vi "Bass Only Live.vi"() -> ()   [LabVIEW 2009]
uses:
  <vilib>/vision/Image Controls.llb/IMAQ Image.ctl
  <vilib>/Instr/_visa.llb/VISA Configure Serial Port (Instr).vi
  <vilib>/userDefined/High Color/IMAQdx.ctl
  <vilib>/Analysis/3filter.llb/Filter Passband Type.ctl
  <vilib>/Analysis/3filter.llb/Butterworth Filter (DBL).vi
  <vilib>/vision/NI_Vision_Development_Module.lvlib
  <vilib>/Analysis/NI_AALBase.lvlib
  <vilib>/vision/driver/NI_Vision_Acquisition_Software.lvlib
panel:
  in  "Orange Guitar":T1={"Global Rectangle"=[220, 302, 227, 392], "Contours"=[{"ID"=enum."External", "Type"=2, "Coordinates"=[226, 391, 220, 302]}]} {"Contours"."Type" items=["No Selection", "Point", "Line", "Rectangle", "Oval", "Polygon", "Freehand Region", "Annulus", "Unused2", "Unused3", "Broken Line", "Freehand Line", "Rotated Rectangle"]}
  in  "Blue Guitar":T1={"Global Rectangle"=[192, 292, 199, 386], "Contours"=[{"ID"=enum."External", "Type"=2, "Coordinates"=[192, 385, 198, 292]}]} {"Contours"."Type" items=["No Selection", "Point", "Line", "Rectangle", "Oval", "Polygon", "Freehand Region", "Annulus", "Unused2", "Unused3", "Broken Line", "Freehand Line", "Rotated Rectangle"]}
  out "Orange Guitar":dbl[](graph)
  out "Orange Guitar LED":bool
  in  "sampling 8":dbl=1.0 format="%0.2f"
  in  "high 9":dbl=60.0 format="%0.2f"
  in  "low  8":dbl=0.12500000000000006 format="%0.4f"
  out "Orange Guitar":T1={"Global Rectangle"=[300, 297, 320, 380], "Contours"=[{"ID"=enum."External", "Type"=2, "Coordinates"=[300, 379, 319, 297]}]} {"Contours"."Type" items=["No Selection", "Point", "Line", "Rectangle", "Oval", "Polygon", "Freehand Region", "Annulus", "Unused2", "Unused3", "Broken Line", "Freehand Line", "Rotated Rectangle"]}
  in  "Green Guitar":T1={"Global Rectangle"=[100, 292, 131, 371], "Contours"=[{"ID"=enum."External", "Type"=2, "Coordinates"=[100, 370, 130, 292]}]} {"Contours"."Type" items=["No Selection", "Point", "Line", "Rectangle", "Oval", "Polygon", "Freehand Region", "Annulus", "Unused2", "Unused3", "Broken Line", "Freehand Line", "Rotated Rectangle"]}
  in  "Red Guitar":T1={"Global Rectangle"=[129, 294, 154, 376], "Contours"=[{"ID"=enum."External", "Type"=2, "Coordinates"=[129, 375, 153, 294]}]} {"Contours"."Type" items=["No Selection", "Point", "Line", "Rectangle", "Oval", "Polygon", "Freehand Region", "Annulus", "Unused2", "Unused3", "Broken Line", "Freehand Line", "Rotated Rectangle"]}
  in  "Yellow Guitar":T1={"Global Rectangle"=[160, 295, 175, 378], "Contours"=[{"ID"=enum."External", "Type"=2, "Coordinates"=[160, 377, 174, 295]}]} {"Contours"."Type" items=["No Selection", "Point", "Line", "Rectangle", "Oval", "Polygon", "Freehand Region", "Annulus", "Unused2", "Unused3", "Broken Line", "Freehand Line", "Rotated Rectangle"]}
  in  "sampling  8":dbl=1.0 format="%0.2f"
  in  "high 8":dbl=60.0 format="%0.2f"
  out "Blue Guitar":dbl[](graph)
  in  "low 2":dbl=0.12500000000000006 format="%0.4f"
  out "Yellow Guitar":dbl[](graph)
  out "Yellow Guitar LED":bool
  in  "sampling 7":dbl=1.0 format="%0.2f"
  in  "high 7":dbl=60.0 format="%0.2f"
  in  "low  7":dbl=0.12500000000000006 format="%0.4f"
  out "Yellow Guitar":T1={"Global Rectangle"=[243, 262, 261, 384], "Contours"=[{"ID"=enum."External", "Type"=2, "Coordinates"=[260, 383, 243, 262]}]} {"Contours"."Type" items=["No Selection", "Point", "Line", "Rectangle", "Oval", "Polygon", "Freehand Region", "Annulus", "Unused2", "Unused3", "Broken Line", "Freehand Line", "Rotated Rectangle"]}
  out "Blue Guitar":T1={"Global Rectangle"=[168, 264, 180, 378], "Contours"=[{"ID"=enum."External", "Type"=2, "Coordinates"=[168, 377, 179, 264]}]} {"Contours"."Type" items=["No Selection", "Point", "Line", "Rectangle", "Oval", "Polygon", "Freehand Region", "Annulus", "Unused2", "Unused3", "Broken Line", "Freehand Line", "Rotated Rectangle"]}
  out "Green Guitar":dbl[](graph)
  out "Green Guitar LED":bool
  in  "sampling 6":dbl=1.0 format="%0.2f"
  in  "high 6":dbl=60.0 format="%0.2f"
  in  "low  6":dbl=0.12500000000000006 format="%0.4f"
  out "Green Guitar":T1={"Global Rectangle"=[406, 309, 423, 383], "Contours"=[{"ID"=enum."External", "Type"=2, "Coordinates"=[422, 382, 406, 309]}]} {"Contours"."Type" items=["No Selection", "Point", "Line", "Rectangle", "Oval", "Polygon", "Freehand Region", "Annulus", "Unused2", "Unused3", "Broken Line", "Freehand Line", "Rotated Rectangle"]}
  out "Red Guitar":dbl[](graph)
  out "Red Guitar LED":bool
  in  "sampling 5":dbl=1.0 format="%0.2f"
  in  "high 5":dbl=60.0 format="%0.2f"
  in  "low  5":dbl=0.12500000000000006 format="%0.4f"
  out "Red Guitar":T1={"Global Rectangle"=[300, 297, 320, 380], "Contours"=[{"ID"=enum."External", "Type"=2, "Coordinates"=[300, 379, 319, 297]}]} {"Contours"."Type" items=["No Selection", "Point", "Line", "Rectangle", "Oval", "Polygon", "Freehand Region", "Annulus", "Unused2", "Unused3", "Broken Line", "Freehand Line", "Rotated Rectangle"]}
  out "Blue Guitar LED":bool
  in  "Mask":T1 {"Contours"."Type" items=["No Selection", "Point", "Line", "Rectangle", "Oval", "Polygon", "Freehand Region", "Annulus", "Unused2", "Unused3", "Broken Line", "Freehand Line", "Rotated Rectangle"]}
  out "Image 2":T2(plugin-control)
  out "Red Line":T1={"Global Rectangle"=[300, 297, 320, 380], "Contours"=[{"ID"=enum."External", "Type"=2, "Coordinates"=[300, 379, 319, 297]}]} {"Contours"."Type" items=["No Selection", "Point", "Line", "Rectangle", "Oval", "Polygon", "Freehand Region", "Annulus", "Unused2", "Unused3", "Broken Line", "Freehand Line", "Rotated Rectangle"]}
  in  "Red Line":T1={"Global Rectangle"=[300, 297, 320, 380], "Contours"=[{"ID"=enum."External", "Type"=2, "Coordinates"=[300, 379, 319, 297]}]} {"Contours"."Type" items=["No Selection", "Point", "Line", "Rectangle", "Oval", "Polygon", "Freehand Region", "Annulus", "Unused2", "Unused3", "Broken Line", "Freehand Line", "Rotated Rectangle"]}
  out "Waveform Red":dbl[](graph)
  out "LED Red":bool
  in  "sampling 4":dbl=1.0 format="%0.2f"
  in  "high 4":dbl=60.0 format="%0.2f"
  in  "low  4":dbl=0.12500000000000006 format="%0.4f"
  out "Green Line":T1={"Global Rectangle"=[406, 309, 423, 383], "Contours"=[{"ID"=enum."External", "Type"=2, "Coordinates"=[422, 382, 406, 309]}]} {"Contours"."Type" items=["No Selection", "Point", "Line", "Rectangle", "Oval", "Polygon", "Freehand Region", "Annulus", "Unused2", "Unused3", "Broken Line", "Freehand Line", "Rotated Rectangle"]}
  in  "Blue Line":T1={"Global Rectangle"=[374, 278, 383, 377], "Contours"=[{"ID"=enum."External", "Type"=2, "Coordinates"=[382, 376, 374, 278]}]} {"Contours"."Type" items=["No Selection", "Point", "Line", "Rectangle", "Oval", "Polygon", "Freehand Region", "Annulus", "Unused2", "Unused3", "Broken Line", "Freehand Line", "Rotated Rectangle"]}
  in  "Green Line":T1={"Global Rectangle"=[406, 309, 423, 383], "Contours"=[{"ID"=enum."External", "Type"=2, "Coordinates"=[422, 382, 406, 309]}]} {"Contours"."Type" items=["No Selection", "Point", "Line", "Rectangle", "Oval", "Polygon", "Freehand Region", "Annulus", "Unused2", "Unused3", "Broken Line", "Freehand Line", "Rotated Rectangle"]}
  in  "low  3":dbl=0.12500000000000006 format="%0.4f"
  out "Waveform Green":dbl[](graph)
  out "LED Green":bool
  in  "sampling 3":dbl=1.0 format="%0.2f"
  in  "high 3":dbl=60.0 format="%0.2f"
  in  "Yellow Line":T1={"Global Rectangle"=[342, 292, 349, 377], "Contours"=[{"ID"=enum."External", "Type"=2, "Coordinates"=[342, 376, 348, 292]}]} {"Contours"."Type" items=["No Selection", "Point", "Line", "Rectangle", "Oval", "Polygon", "Freehand Region", "Annulus", "Unused2", "Unused3", "Broken Line", "Freehand Line", "Rotated Rectangle"]}
  out "Blue Line":T1={"Global Rectangle"=[168, 264, 180, 378], "Contours"=[{"ID"=enum."External", "Type"=2, "Coordinates"=[168, 377, 179, 264]}]} {"Contours"."Type" items=["No Selection", "Point", "Line", "Rectangle", "Oval", "Polygon", "Freehand Region", "Annulus", "Unused2", "Unused3", "Broken Line", "Freehand Line", "Rotated Rectangle"]}
  out "cluster":T3
  in  "baud rate (9600)":u32=9600
  in  "VISA resource name":refnum<visa-resource-name>
  out "number":u8
  out "decimal integer string":string
  out "Image Dst Out":T2
  out "Yellow Line":T1={"Global Rectangle"=[243, 262, 261, 384], "Contours"=[{"ID"=enum."External", "Type"=2, "Coordinates"=[260, 383, 243, 262]}]} {"Contours"."Type" items=["No Selection", "Point", "Line", "Rectangle", "Oval", "Polygon", "Freehand Region", "Annulus", "Unused2", "Unused3", "Broken Line", "Freehand Line", "Rotated Rectangle"]}
  in  "low  2":dbl=0.12500000000000006 format="%0.4f"
  in  "high 2":dbl=60.0 format="%0.2f"
  in  "sampling 2":dbl=1.0 format="%0.2f"
  out "LED Yellow":bool
  out "Waveform Yellow":dbl[](graph)
  in  "playtime":dbl=30.0
  out "Frame Number":i32
  in  "Frame Start":i32=2400
  out "Blue Drum":bool
  in  "low":dbl=0.12500000000000006 format="%0.4f"
  out "Blue Drum":dbl[](graph)
  in  "high":dbl=60.0 format="%0.2f"
  in  "sampling":dbl=1.0 format="%0.2f"
  in  "stop":bool
  # "BLUE"
  # "YELLOW"
  # "GREEN"
  # "RED"
  # "Drums"
  # "Guitar"
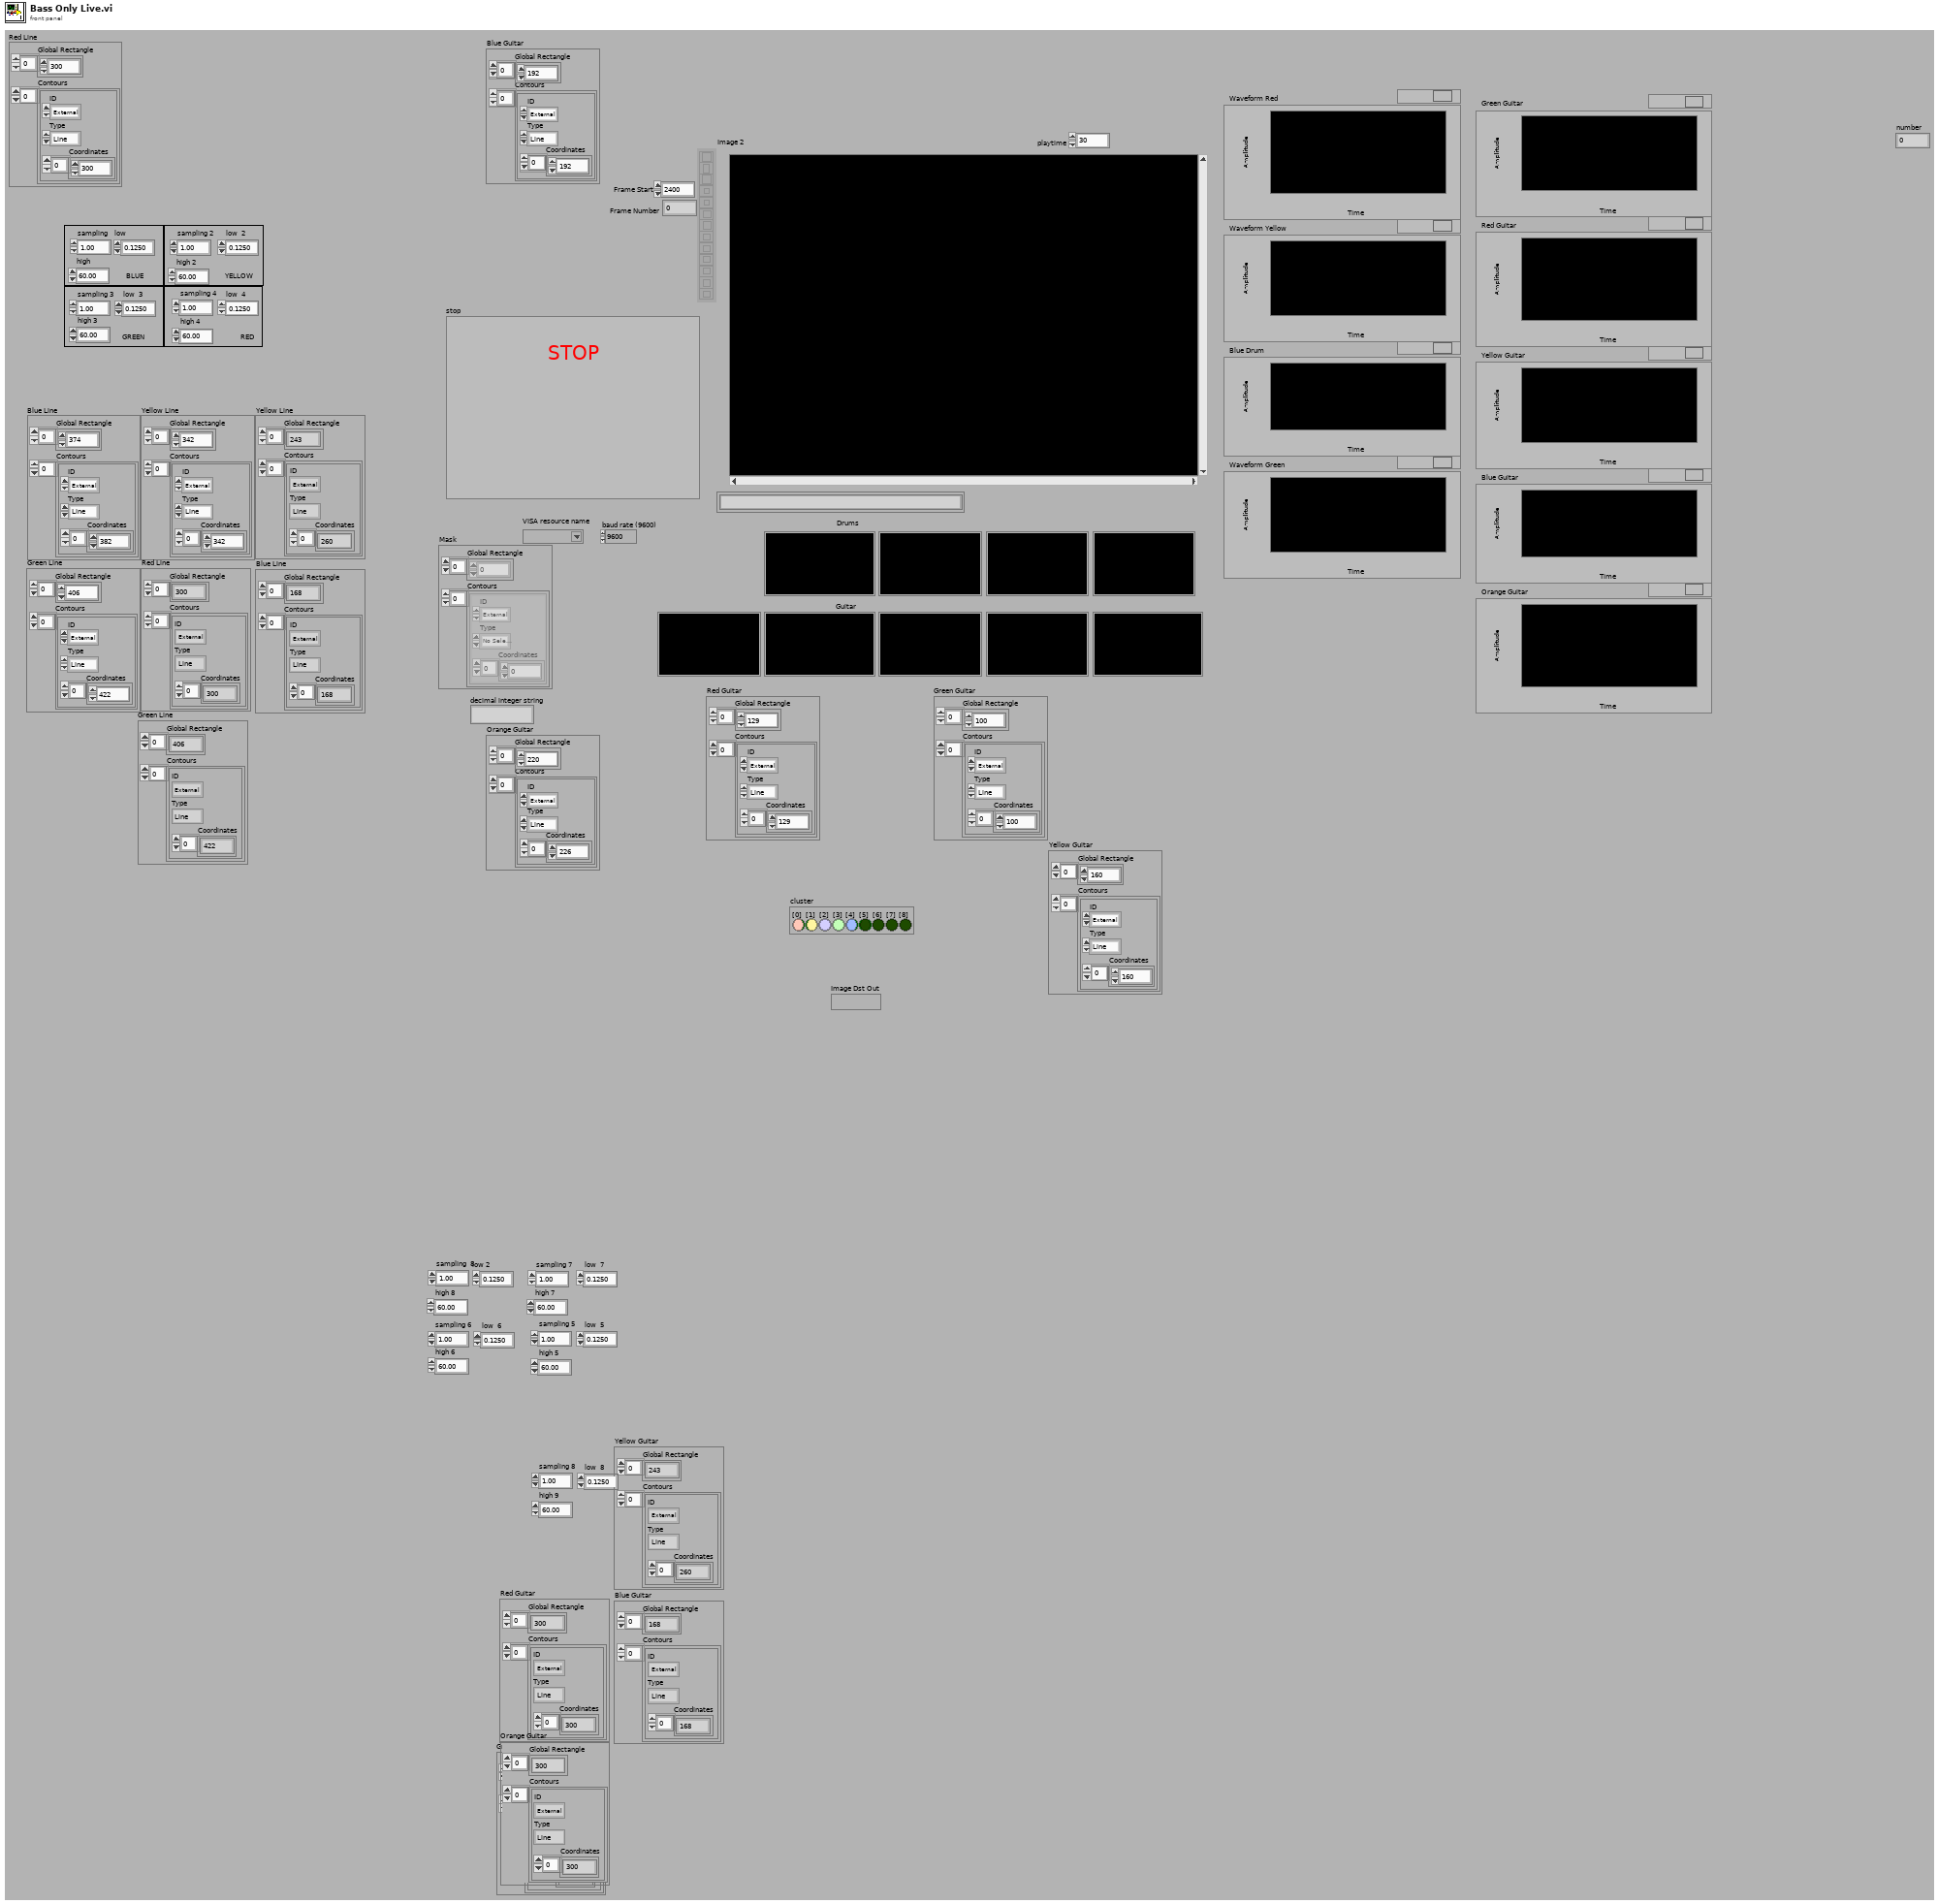
[diagram p1: front panel]
types:
  T1 = cluster{"Global Rectangle":i32[], "Contours":cluster{"ID":enum32{"External", "Internal"}, "Type":u32, "Coordinates":i32[]}[]}
  T2 = typedef "IMAQ Image.ctl" = refnum<image>
  T3 = cluster{"[0]":bool, "[1]":bool, "[2]":bool, "[3]":bool, "[4]":bool, "[5]":bool, "[6]":bool, "[7]":bool, "[8]":bool}
  T4 = typedef "IMAQdx.ctl" = refnum<k21>
  T5 = typedef "NI_AALBase.lvlib/Filter Passband Type.ctl" = enum32{"Lowpass", "Highpass", "Bandpass", "Bandstop"}
  T6 = cluster{"Left":i32, "Top":i32, "Right":i32, "Bottom":i32}
  T7 = typedef "Image Type" = u32
  T8 = cluster{"ID":enum32{"External", "Internal"}, "Type":u32, "Coordinates":i32[]}[]
  T9 = cluster{"ID":enum32{"External", "Internal"}, "Type":u32, "Coordinates":i32[]}
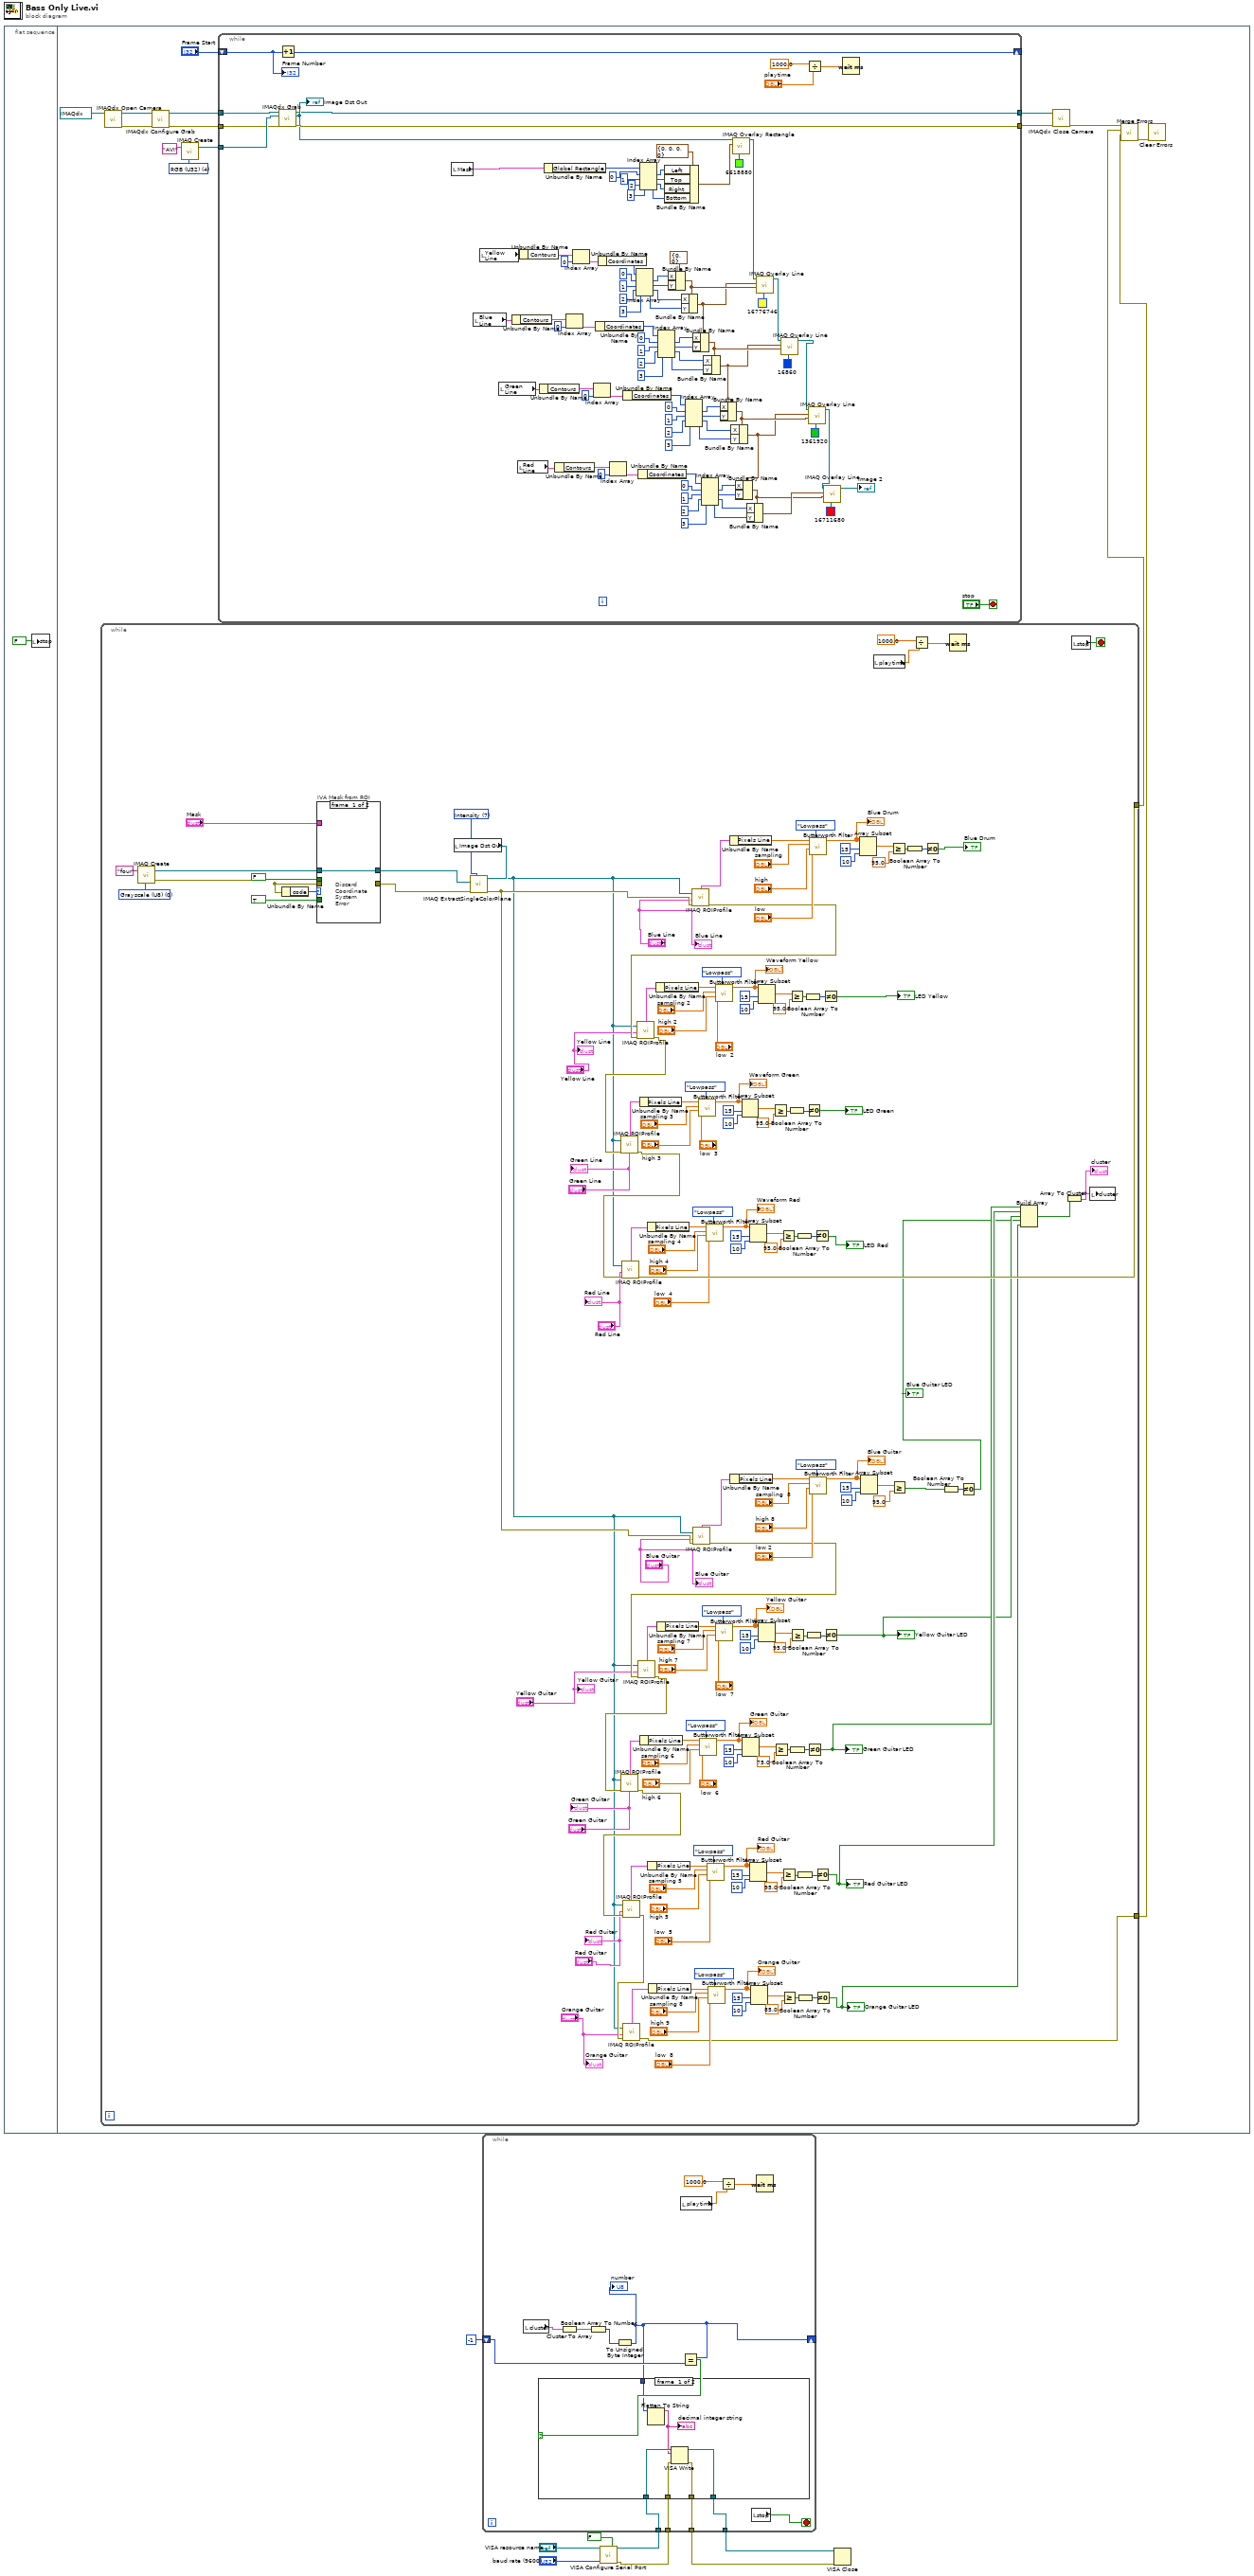
[diagram p0: block diagram]
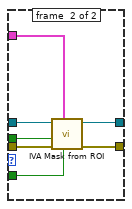
[diagram p3: hidden frame]
diagram:
  n1 = flat-sequence {
    frame #0 {
      n2 = local write "stop"(FALSE ("stop")) -> ()
    }
    frame #1 {
      w22 = T7 4 items=["Grayscale (U8)", "Grayscale (I16)", "Grayscale (SGL)", "Complex (CSG)", "RGB (U32)", "HSL (U32)", "RGB (U64)", "Grayscale (U16)"] ("Image Type")
      n3 = while {
        tunnel: [w172] -> w19
        tunnel: [w39] -> w18
        stop <- w187 stop-if-true
        w182 = T7 0 items=["Grayscale (U8)", "Grayscale (I16)", "Grayscale (SGL)", "Complex (CSG)", "RGB (U32)", "HSL (U32)", "RGB (U64)", "Grayscale (U16)"] ("Image Type")
        w188 = 7 items=["Red", "Green", "Blue", "Hue", "Saturation", "Luminance", "Value", "Intensity"] ("Color Plane")
        n4 = call "IMAQ Create"("Image Name"="four", "Image Type"=w182) -> ("New Image"=w175:T2, "error out"=w176:errorcluster)  [unwired: 3 in]
        n5 = Unbundle By Name(w176) -> ("code"=w180:i32)
        n6 = case "IVA Mask from ROI" shown="Default" w180 {
          tunnel: "Mask" -> [_ w196]
          tunnel: TRUE ("Shrink") -> [_ w195]
          tunnel: w175 -> [w189 w194]
          tunnel: w176 -> [_ w193]
          tunnel: [_ w192] -> w177
          tunnel: [w189 w191] -> w173
          tunnel: FALSE ("Out / In") -> [_ w190]
          frame #0 {
            # "Discard\nCoordinate\nSystem\nError"
          }
          frame #1 {
            n7 = call <vilib>:"IVA Mask from ROI.vi"("Shrink"=w195, "ROI Descriptor"=w196, "error in (no error)"=w193, "Out / In"=w190, "Image Src"=w194) -> ("error out"=w192:errorcluster, "Image Out"=w191:T2)  [unwired: 5 out]
          }
        }
        n8 = local read "Image Dst Out"() -> (w183:T2)
        n9 = call "IMAQ ExtractSingleColorPlane"("Color Plane"=w188, "error in (no error)"=w177, "Image Dst"=w173, "Image Src"=w183) -> ("error out"=w171:errorcluster, "Image Dst Out"=w38:T2)  [unwired: 6 out]
        n10 = call "IMAQ ROIProfile"("error in (no error)"=w171, "ROI Descriptor"="Blue Line", "Image"=w38) -> ("error out"=w146:errorcluster, "ROI Graph"=w145:cluster{"x0":sgl, "dx":sgl, "Pixels Line":sgl[]})  [unwired: 4 out]
        n11 = call "IMAQ ROIProfile"("error in (no error)"=w146, "ROI Descriptor"="Yellow Line", "Image"=w38) -> ("error out"=w113:errorcluster, "ROI Graph"=w149:cluster{"x0":sgl, "dx":sgl, "Pixels Line":sgl[]})  [unwired: 4 out]
        n12 = call "IMAQ ROIProfile"("error in (no error)"=w113, "ROI Descriptor"="Green Line", "Image"=w38) -> ("error out"=w116:errorcluster, "ROI Graph"=w143:cluster{"x0":sgl, "dx":sgl, "Pixels Line":sgl[]})  [unwired: 4 out]
        n13 = call "IMAQ ROIProfile"("error in (no error)"=w116, "ROI Descriptor"="Red Line", "Image"=w38) -> ("error out"=w172:errorcluster, "ROI Graph"=w118:cluster{"x0":sgl, "dx":sgl, "Pixels Line":sgl[]})  [unwired: 4 out]
        n14 = Unbundle By Name(w143) -> ("Pixels Line"=w140:sgl[])
        n15 = Unbundle By Name(w118) -> ("Pixels Line"=w121:sgl[])
        n16 = Unbundle By Name(w149) -> ("Pixels Line"=w152:sgl[])
        n17 = call "IMAQ ROIProfile"("error in (no error)"=w171, "ROI Descriptor"="Blue Guitar", "Image"=w38) -> ("error out"=w87:errorcluster, "ROI Graph"=w86:cluster{"x0":sgl, "dx":sgl, "Pixels Line":sgl[]})  [unwired: 4 out]
        n18 = call "IMAQ ROIProfile"("error in (no error)"=w87, "ROI Descriptor"="Yellow Guitar", "Image"=w38) -> ("error out"=w57:errorcluster, "ROI Graph"=w90:cluster{"x0":sgl, "dx":sgl, "Pixels Line":sgl[]})  [unwired: 4 out]
        n19 = call "IMAQ ROIProfile"("error in (no error)"=w57, "ROI Descriptor"="Green Guitar", "Image"=w38) -> ("error out"=w58:errorcluster, "ROI Graph"=w84:cluster{"x0":sgl, "dx":sgl, "Pixels Line":sgl[]})  [unwired: 4 out]
        n20 = call "IMAQ ROIProfile"("error in (no error)"=w58, "ROI Descriptor"="Red Guitar", "Image"=w38) -> ("error out"=w40:errorcluster, "ROI Graph"=w60:cluster{"x0":sgl, "dx":sgl, "Pixels Line":sgl[]})  [unwired: 4 out]
        n21 = call "IMAQ ROIProfile"("error in (no error)"=w40, "ROI Descriptor"="Orange Guitar", "Image"=w38) -> ("error out"=w39:errorcluster, "ROI Graph"=w52:cluster{"x0":sgl, "dx":sgl, "Pixels Line":sgl[]})  [unwired: 4 out]
        n22 = Unbundle By Name(w84) -> ("Pixels Line"=w81:sgl[])
        n23 = Unbundle By Name(w60) -> ("Pixels Line"=w63:sgl[])
        n24 = Unbundle By Name(w52) -> ("Pixels Line"=w49:sgl[])
        n25 = Unbundle By Name(w90) -> ("Pixels Line"=w93:sgl[])
        n26 = call-poly <vilib>:"Butterworth Filter.vi"("filter type"=Filter_Passband_Type."Lowpass", "low cutoff freq: fl"="low  3", "high cutoff freq: fh"="high 3", "sampling freq: fs"="sampling 3", "X"=w140) -> ("Filtered X"=w144:dbl[])  [unwired: 3 in, 1 out]
        "Waveform Green" <- w144
        n27 = call-poly <vilib>:"Butterworth Filter.vi"("filter type"=Filter_Passband_Type."Lowpass", "low cutoff freq: fl"="low  6", "high cutoff freq: fh"="high 6", "sampling freq: fs"="sampling 6", "X"=w81) -> ("Filtered X"=w85:dbl[])  [unwired: 3 in, 1 out]
        "Green Guitar" <- w85
        n28 = call-poly <vilib>:"Butterworth Filter.vi"("filter type"=Filter_Passband_Type."Lowpass", "low cutoff freq: fl"="low  4", "high cutoff freq: fh"="high 4", "sampling freq: fs"="sampling 4", "X"=w121) -> ("Filtered X"=w117:dbl[])  [unwired: 3 in, 1 out]
        "Waveform Red" <- w117
        n29 = call-poly <vilib>:"Butterworth Filter.vi"("filter type"=Filter_Passband_Type."Lowpass", "low cutoff freq: fl"="low  5", "high cutoff freq: fh"="high 5", "sampling freq: fs"="sampling 5", "X"=w63) -> ("Filtered X"=w59:dbl[])  [unwired: 3 in, 1 out]
        "Red Guitar" <- w59
        n30 = call-poly <vilib>:"Butterworth Filter.vi"("filter type"=Filter_Passband_Type."Lowpass", "low cutoff freq: fl"="low  8", "high cutoff freq: fh"="high 9", "sampling freq: fs"="sampling 8", "X"=w49) -> ("Filtered X"=w53:dbl[])  [unwired: 3 in, 1 out]
        "Orange Guitar" <- w53
        n31 = call-poly <vilib>:"Butterworth Filter.vi"("filter type"=Filter_Passband_Type."Lowpass", "low cutoff freq: fl"="low  2", "high cutoff freq: fh"="high 2", "sampling freq: fs"="sampling 2", "X"=w152) -> ("Filtered X"=w148:dbl[])  [unwired: 3 in, 1 out]
        "Waveform Yellow" <- w148
        n32 = call-poly <vilib>:"Butterworth Filter.vi"("filter type"=Filter_Passband_Type."Lowpass", "low cutoff freq: fl"="low  7", "high cutoff freq: fh"="high 7", "sampling freq: fs"="sampling 7", "X"=w93) -> ("Filtered X"=w89:dbl[])  [unwired: 3 in, 1 out]
        "Yellow Guitar" <- w89
        n33 = Unbundle By Name(w145) -> ("Pixels Line"=w169:sgl[])
        n34 = Unbundle By Name(w86) -> ("Pixels Line"=w109:sgl[])
        n35 = Array Subset(array=w144, index=15, length=10) -> (w135:dbl[])
        n36 = Array Subset(array=w85, index=15, length=10) -> (w76:dbl[])
        n37 = Array Subset(array=w117, index=15, length=10) -> (w126:dbl[])
        n38 = Array Subset(array=w59, index=15, length=10) -> (w68:dbl[])
        n39 = Array Subset(array=w53, index=15, length=10) -> (w44:dbl[])
        n40 = Array Subset(array=w148, index=15, length=10) -> (w157:dbl[])
        n41 = Array Subset(array=w89, index=15, length=10) -> (w98:dbl[])
        n42 = Greater Or Equal?(x=w135, y=95.0) -> (x >= y?=w137:bool[])
        n43 = Greater Or Equal?(x=w76, y=75.0) -> (x >= y?=w78:bool[])
        n44 = Greater Or Equal?(x=w126, y=95.0) -> (x >= y?=w124:bool[])
        n45 = Greater Or Equal?(x=w68, y=95.0) -> (x >= y?=w66:bool[])
        n46 = Greater Or Equal?(x=w44, y=85.0) -> (x >= y?=w46:bool[])
        n47 = Boolean Array To Number(Boolean array=w137) -> (number=w138:u32)
        n48 = Greater Or Equal?(x=w157, y=95.0) -> (x >= y?=w155:bool[])
        n49 = Boolean Array To Number(Boolean array=w78) -> (number=w79:u32)
        n50 = Greater Or Equal?(x=w98, y=95.0) -> (x >= y?=w96:bool[])
        n51 = Boolean Array To Number(Boolean array=w124) -> (number=w123:u32)
        n52 = Boolean Array To Number(Boolean array=w66) -> (number=w65:u32)
        n53 = Boolean Array To Number(Boolean array=w46) -> (number=w47:u32)
        n54 = Boolean Array To Number(Boolean array=w155) -> (number=w154:u32)
        n55 = Boolean Array To Number(Boolean array=w96) -> (number=w95:u32)
        n56 = Not Equal To 0?(x=w138) -> (x != 0?=→"LED Green":bool)
        n57 = Not Equal To 0?(x=w79) -> (x != 0?=w32:bool)
        "Green Guitar LED" <- w32
        n58 = call-poly <vilib>:"Butterworth Filter.vi"("filter type"=Filter_Passband_Type."Lowpass", "low cutoff freq: fl"="low", "high cutoff freq: fh"="high", "sampling freq: fs"="sampling", "X"=w169) -> ("Filtered X"=w131:dbl[])  [unwired: 3 in, 1 out]
        "Blue Drum" <- w131
        n59 = call-poly <vilib>:"Butterworth Filter.vi"("filter type"=Filter_Passband_Type."Lowpass", "low cutoff freq: fl"="low 2", "high cutoff freq: fh"="high 8", "sampling freq: fs"="sampling  8", "X"=w109) -> ("Filtered X"=w72:dbl[])  [unwired: 3 in, 1 out]
        "Blue Guitar" <- w72
        n60 = Not Equal To 0?(x=w123) -> (x != 0?=→"LED Red":bool)
        n61 = Not Equal To 0?(x=w65) -> (x != 0?=w31:bool)
        "Red Guitar LED" <- w31
        n62 = Not Equal To 0?(x=w47) -> (x != 0?=w28:bool)
        "Orange Guitar LED" <- w28
        n63 = Not Equal To 0?(x=w154) -> (x != 0?=→"LED Yellow":bool)
        n64 = Not Equal To 0?(x=w95) -> (x != 0?=w30:bool)
        "Yellow Guitar LED" <- w30
        n65 = Array Subset(array=w131, index=15, length=10) -> (w163:dbl[])
        n66 = Array Subset(array=w72, index=15, length=10) -> (w103:dbl[])
        n67 = local read "playtime"() -> (w184:dbl)
        n68 = Greater Or Equal?(x=w163, y=95.0) -> (x >= y?=w161:bool[])
        n69 = Greater Or Equal?(x=w103, y=95.0) -> (x >= y?=w37:bool[])
        n70 = Boolean Array To Number(Boolean array=w161) -> (number=w160:u32)
        n71 = Divide(x=1000.0, y=w184) -> (x/y=w186:dbl)
        n72 = Not Equal To 0?(x=w160) -> (x != 0?=→"Blue Drum":bool)
        n73 = Boolean Array To Number(Boolean array=w37) -> (number=w101:u32)
        n74 = Wait (ms)(milliseconds to wait=w186) -> ()  [unwired: 1 out]
        n75 = Not Equal To 0?(x=w101) -> (x != 0?=w29:bool)
        "Blue Guitar LED" <- w29
        n76 = Build Array(w32, w31, w30, w29, w28) -> (w112:bool[])
        n77 = Array To Cluster(array=w112) -> (cluster=w27:T3)
        "cluster" <- w27
        n78 = local read "stop"() -> (w187:bool)
        n79 = local write "cluster"(w27) -> ()
        "Yellow Line" <- "Yellow Line"
        "Blue Line" <- "Blue Line"
        "Green Line" <- "Green Line"
        "Red Line" <- "Red Line"
        "Yellow Guitar" <- "Yellow Guitar"
        "Blue Guitar" <- "Blue Guitar"
        "Green Guitar" <- "Green Guitar"
        "Red Guitar" <- "Red Guitar"
        "Orange Guitar" <- "Orange Guitar"
      }
      n80 = call <vilib>:"IMAQdx Open Camera.vi"("Session In"=T4 "cam1") -> ("error out"=w17:errorcluster, "Session Out"=w16:T4)  [unwired: 9 in]
      n81 = call <vilib>:"IMAQdx Configure Grab.vi"("error in"=w17, "Session In"=w16) -> ("error out"=w13:errorcluster, "Session Out"=w14:T4)  [unwired: 8 in]
      n82 = call "IMAQ Create"("Image Name"="AVI", "Image Type"=w22) -> ("New Image"=w20:T2)  [unwired: 3 in, 1 out]
      n83 = while {
        tunnel: w14 -> [w200]
        tunnel: w13 -> [w199]
        tunnel: [w197] -> w10
        shift-right: [w287] -> _
        shift-left: "Frame Start" -> [w286]
        tunnel: [w202] -> w11
        tunnel: w20 -> [w201]
        stop <- "stop" stop-if-true
        n84 = call <vilib>:"IMAQdx Grab.vi"("error in"=w199, "Image In"=w201, "Session In"=w200) -> ("error out"=w202:errorcluster, "Image Out"=w198:T2, "Session Out"=w197:T4)  [unwired: 5 in, 1 out]
        "Image Dst Out" <- w198
        n85 = Increment(x=w286) -> (x+1=w287:i32)
        n86 = local read "Mask"() -> (w203:T1)
        n87 = local read "Blue Line"() -> (w241:T1)
        n88 = local read "Yellow Line"() -> (w240:T1)
        n89 = local read "Green Line"() -> (w239:T1)
        n90 = Unbundle By Name(w241) -> ("Contours"=w253:T8)
        n91 = local read "Red Line"() -> (w206:T1)
        n92 = Unbundle By Name(w240) -> ("Contours"=w268:T8)
        n93 = Unbundle By Name(w239) -> ("Contours"=w229:T8)
        n94 = Unbundle By Name(w203) -> ("Global Rectangle"=w282:i32[])
        n95 = Unbundle By Name(w206) -> ("Contours"=w216:T8)
        n96 = Index Array(array=w253, index=0) -> (element=w252:T9)
        n97 = Index Array(array=w268, index=0) -> (element=w270:T9)
        n98 = Index Array(array=w229, index=0) -> (element=w230:T9)
        n99 = Unbundle By Name(w252) -> ("Coordinates"=w251:i32[])
        n100 = Unbundle By Name(w270) -> ("Coordinates"=w271:i32[])
        n101 = Index Array(array=w216, index=0) -> (element=w215:T9)
        n102 = Unbundle By Name(w230) -> ("Coordinates"=w231:i32[])
        n103 = Index Array(array=w271, index #1=0 ("index"), index #2=1 ("index"), index #3=2 ("index"), index #4=3 ("index")) -> (element #1=w263:i32, element #2=w264:i32, element #3=w265:i32, element #4=w266:i32)
        n104 = Unbundle By Name(w215) -> ("Coordinates"=w214:i32[])
        n105 = Index Array(array=w282, index #1=0 ("index"), index #2=1 ("index"), index #3=2 ("index"), index #4=3 ("index")) -> (element #1=w281:i32, element #2=w280:i32, element #3=w279:i32, element #4=w278:i32)
        n106 = Index Array(array=w251, index #1=0 ("index"), index #2=1 ("index"), index #3=2 ("index"), index #4=3 ("index")) -> (element #1=w250:i32, element #2=w256:i32, element #3=w255:i32, element #4=w254:i32)
        n107 = Bundle By Name(cluster=T6 {"Left"=0, "Top"=0, "Right"=0, "Bottom"=0} ("Rectangle"), "Left"=w281, "Top"=w280, "Right"=w279, "Bottom"=w278) -> (w284:T6)
        n108 = Bundle By Name(cluster=cluster{"X":i32, "Y":i32} {"X"=0, "Y"=0} ("End Point"), "X"=w263, "Y"=w264) -> (w272:cluster{"X":i32, "Y":i32})
        n109 = Bundle By Name(cluster=w272, "X"=w265, "Y"=w266) -> (w243:cluster{"X":i32, "Y":i32})
        n110 = Index Array(array=w231, index #1=0 ("index"), index #2=1 ("index"), index #3=2 ("index"), index #4=3 ("index")) -> (element #1=w232:i32, element #2=w226:i32, element #3=w227:i32, element #4=w228:i32)
        n111 = Bundle By Name(cluster=w243, "X"=w250, "Y"=w256) -> (w257:cluster{"X":i32, "Y":i32})
        n112 = Index Array(array=w214, index #1=0 ("index"), index #2=1 ("index"), index #3=2 ("index"), index #4=3 ("index")) -> (element #1=w213:i32, element #2=w219:i32, element #3=w218:i32, element #4=w217:i32)
        n113 = Bundle By Name(cluster=w257, "X"=w255, "Y"=w254) -> (w224:cluster{"X":i32, "Y":i32})
        n114 = Bundle By Name(cluster=w224, "X"=w232, "Y"=w226) -> (w223:cluster{"X":i32, "Y":i32})
        n115 = Bundle By Name(cluster=w223, "X"=w227, "Y"=w228) -> (w205:cluster{"X":i32, "Y":i32})
        n116 = call "IMAQ Overlay Rectangle"("Color"=u32 6618880, "Rectangle"=w284, "Image"=w198) -> ("Image Out"=w258:T2)  [unwired: 7 in, 1 out]
        n117 = Bundle By Name(cluster=w205, "X"=w213, "Y"=w219) -> (w221:cluster{"X":i32, "Y":i32})
        n118 = Bundle By Name(cluster=w221, "X"=w218, "Y"=w217) -> (w222:cluster{"X":i32, "Y":i32})
        n119 = call "IMAQ Overlay Line"("Color"=u32 16776746, "End Point"=w272, "Start Point"=w243, "Image"=w258) -> ("Image Out"=w248:T2)  [unwired: 6 in, 1 out]
        n120 = call "IMAQ Overlay Line"("Color"=u32 16860, "End Point"=w257, "Start Point"=w224, "Image"=w248) -> ("Image Out"=w225:T2)  [unwired: 6 in, 1 out]
        n121 = Divide(x=1000.0, y="playtime") -> (x/y=w290:dbl)
        n122 = call "IMAQ Overlay Line"("Color"=u32 1361920, "End Point"=w223, "Start Point"=w205, "Image"=w225) -> ("Image Out"=w204:T2)  [unwired: 6 in, 1 out]
        n123 = call "IMAQ Overlay Line"("Color"=u32 16711680, "End Point"=w221, "Start Point"=w222, "Image"=w204) -> ("Image Out"=→"Image 2":T2)  [unwired: 6 in, 1 out]
        n124 = Wait (ms)(milliseconds to wait=w290) -> ()  [unwired: 1 out]
        "Frame Number" <- w286
      }
      n125 = call <vilib>:"IMAQdx Close Camera.vi"("error in"=w11, "Session In"=w10) -> ("error out"=w12:errorcluster)  [unwired: 9 in]
      n126 = call <vilib>:"Merge Errors.vi"("error in 3 (no error)"=w18, "error in 2 (no error)"=w19, "error in 1 (no error)"=w12) -> ("error out"=w23:errorcluster)  [unwired: 4 in]
      n127 = call <vilib>:"Clear Errors.vi"("error in (no error)"=w23) -> ()  [unwired: 6 in, 1 out]
    }
  }
  n128 = call-poly "VISA Configure Serial Port"("VISA resource name"="VISA resource name", "Enable Termination\nChar (T)"=FALSE ("Enable Termination\nChar (T)"), "baud rate (9600)"="baud rate (9600)") -> ("VISA resource name out"=w7:refnum<visa-resource-name>, "error out"=w2:errorcluster)  [unwired: 11 in]
  n129 = while {
    shift-right: [w292] -> _
    shift-left: -1 -> [w305]
    tunnel: w7 -> [w303]
    tunnel: [w302] -> w6
    tunnel: w2 -> [w301]
    tunnel: [w300] -> w1
    stop <- w297 stop-if-true
    n130 = local read "cluster"() -> (w298:T3)
    n131 = Cluster To Array(cluster=w298) -> (array=w299:bool[])
    n132 = Boolean Array To Number(Boolean array=w299) -> (number=w293:u32)
    n133 = To Unsigned Byte Integer(number=w293) -> (unsigned 8bit integer=w292:u8)
    "number" <- w292
    n134 = local read "playtime"() -> (w296:dbl)
    n135 = Equal?(x=w292, y=w305) -> (x = y?=w304:bool)
    n136 = case shown="False" w304 {
      tunnel: w303 -> [w311 w313]
      tunnel: [w310 w313] -> w302
      tunnel: w292 -> [w307 _]
      tunnel: w301 -> [w309 w312]
      tunnel: [w308 w312] -> w300
      frame #0 {
        n137 = Flatten To String(anything=w307) -> (data string=w306:string)  [unwired: 3 in, 2 out]
        "decimal integer string" <- w306
        n138 = VISA Write(VISA resource name=w311, write buffer=w306, error in (no error)=w309) -> (VISA resource name out=w310:refnum<visa-resource-name>, error out=w308:errorcluster)  [unwired: 1 out]
      }
      frame #1 {
      }
    }
    n139 = Divide(x=1000.0, y=w296) -> (x/y=w294:dbl)
    n140 = local read "stop"() -> (w297:bool)
    n141 = Wait (ms)(milliseconds to wait=w294) -> ()  [unwired: 1 out]
  }
  n142 = VISA Close(VISA resource name=w6, error in (no error)=w1) -> ()  [unwired: 1 out]
